vi "averaged_stokes_acquisition_single_tiff.vi"(0 "Motor \"Name\"":string="1", 1 "Beam Type":string="save_array_as_tiff", 2 "VISA resource name":refnum<visa-resource-name>="COM3", 5 "Encoder Pulses per Degree":i32=398, 7 "Number of Angles":i32=8, 9 "Number of Measures":i32=10, 11 "ICImagingControl In":refnum<k7>, 12 "session in":refnum<k35>, 13 "Saving Path":path=path "C:/Users/Usuario/OneDrive - Universitat de Barcelona/PhD", 14 "module path":path) -> ()   [LabVIEW 2025]
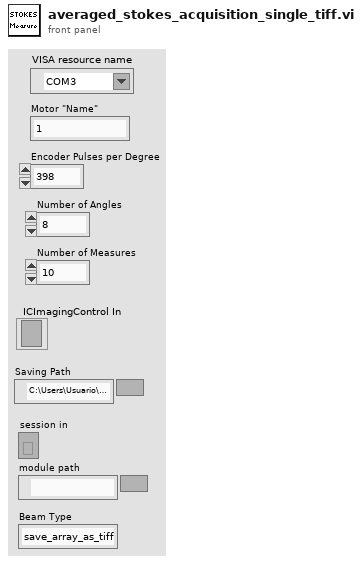
[diagram p1: front panel]
types:
  T1 = typedef "IMAQ Image.ctl" = refnum<image>
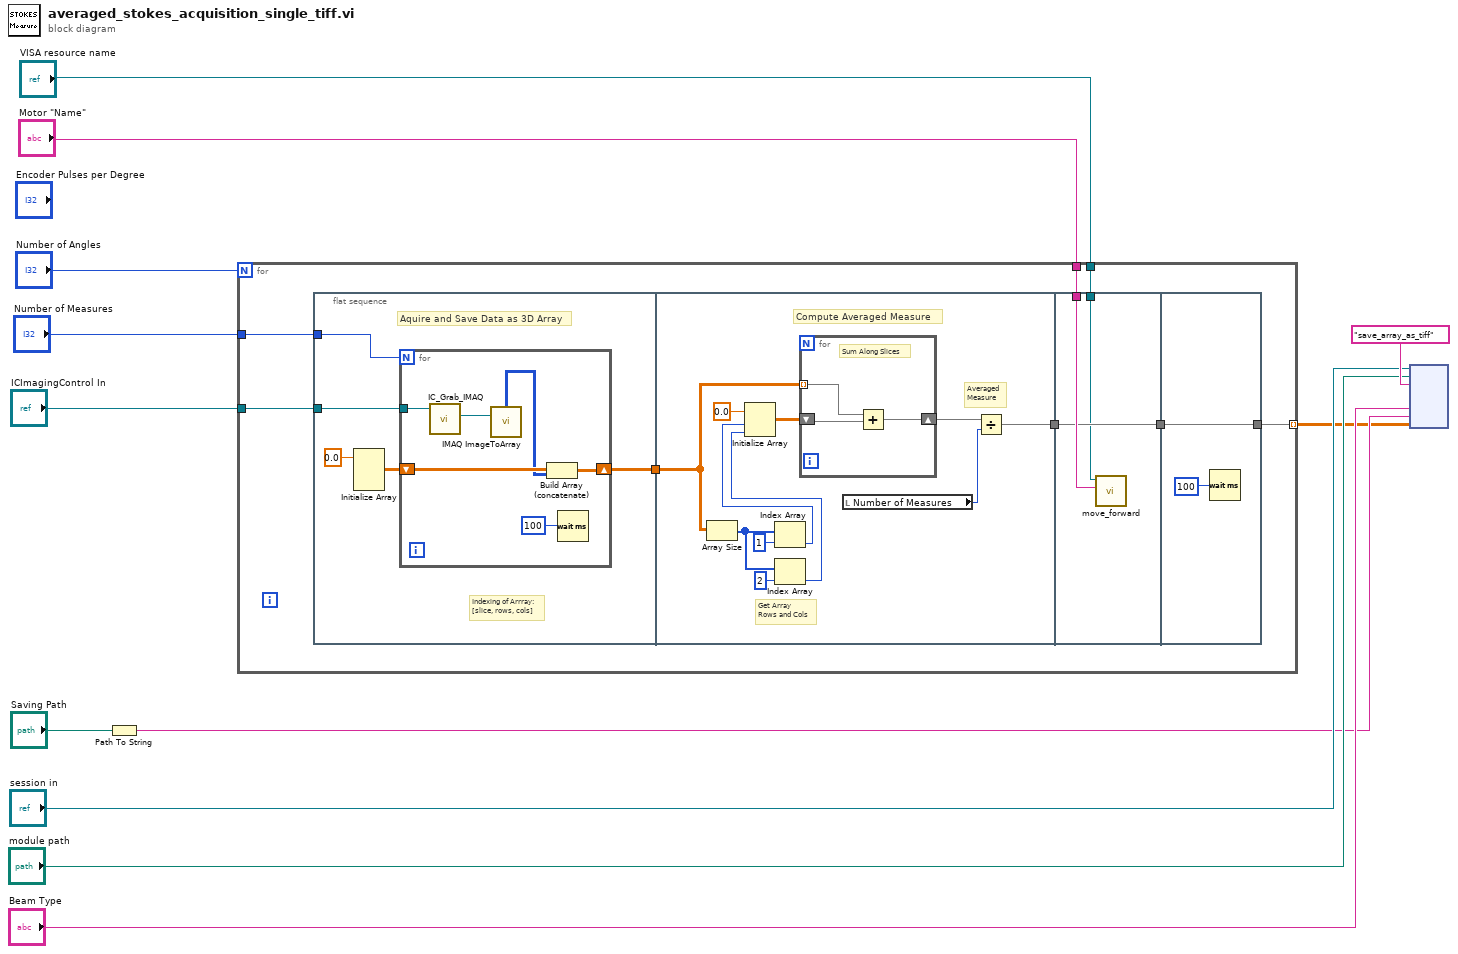
[diagram p0: block diagram]
diagram:
  n1 = Path To String(path="Saving Path") -> (string=w3:string)
  n2 = for {
    N: "Number of Angles" -> [_]
    tunnel: "ICImagingControl In" -> [w20]
    tunnel: "Number of Measures" -> [w19]
    tunnel: "Motor \"Name\"" -> [w17]
    tunnel: [w16] -> w2 mode=indexing
    tunnel: "VISA resource name" -> [w13]
    n3 = flat-sequence {
      tunnel: w20 -> [w25]
      tunnel: w19 -> [w23]
      tunnel: [w22] -> w18
      tunnel: w18 -> [w36]
      tunnel: [w32] -> w14
      tunnel: w17 -> [w48]
      tunnel: [w47] -> w15
      tunnel: w14 -> [w47]
      tunnel: w13 -> [w46]
      tunnel: [w49] -> w16
      tunnel: w15 -> [w49]
      frame #0 {
        # "Aquire and Save Data as 3D Array"
        # "Indexing of Arrray:\n[slice, rows, cols]"
        n4 = Initialize Array(0.0) -> (w24:dbl[][][])  [unwired: 3 in]
        n5 = for {
          N: w23 -> [_]
          tunnel: w25 -> [w29]
          shift-right: [w26] -> w22
          shift-left: w24 -> [w30]
          n6 = call <userlib>:"IC_Grab_IMAQ.vi"("ICImagingControl In"=w29) -> ("Image Out"=w28:T1)  [unwired: 2 in, 3 out]
          n7 = call "IMAQ ImageToArray"("Image"=w28) -> ("Image Pixels (U8)"=w27:u8[][])  [unwired: 3 in, 4 out]
          n8 = Build Array (concatenate)(w30, w27) -> (w26:dbl[][][])
          n9 = Wait (ms)(milliseconds to wait=u32 100) -> ()  [unwired: 1 out]
        }
      }
      frame #1 {
        # "Compute Averaged Measure"
        # "Averaged\nMeasure"
        # "Get Array \nRows and Cols"
        n10 = Array Size(array=w36) -> (size(s)=w41:i32[])
        n11 = Index Array(array=w41, index=1) -> (element=w38:i32)
        n12 = Index Array(array=w41, index=2) -> (element=w37:i32)
        n13 = Initialize Array(0.0 ("element"), w38, w37) -> (w35:dbl[][])
        n14 = for {
          tunnel: w36 -> [w44] mode=indexing
          shift-right: [w43] -> w34
          shift-left: w35 -> [w45]
          # "Sum Along Slices"
          n15 = Add(x=w44, y=w45) -> (x+y=w43:dbl[][])
        }
        n16 = local read "Number of Measures"() -> (w33:i32)
        n17 = Divide(x=w34, y=w33) -> (x/y=w32:dbl[][])
      }
      frame #2 {
        n18 = call "move_forward.vi"("Motor \"Name\""=w48, "VISA resource name"=w46) -> ()  [unwired: 8 in, 2 out]
      }
      frame #3 {
        n19 = Wait (ms)(milliseconds to wait=u32 100) -> ()  [unwired: 1 out]
      }
    }
  }
  n20 = node("session in", "module path", "save_array_as_tiff", "Beam Type", w3, w2) -> ()  [unwired: 6 in, 4 out]
